vi "Retrieve All Paragraphs.vi"(8 "error in (no error)":errorcluster, 11 "xwpfReader in":refnum<class "xwpfReader.lvclass">) -> (0 "error out":errorcluster, 1 "Paragraph Styles":refnum<class "Style.lvclass">[](array[class]), 2 "Paragraphs":string[](array[string]), 3 "xwpfReader out":refnum<class "xwpfReader.lvclass">)   [LabVIEW 2017, in "LabVIEW NPOI.lvlib" / "xwpfReader.lvclass"]
doc: "Retrieves all the Paragraph content from the document. \n\nThis VI iterates through each paragraph to get their contents."
uses:
  xwpfReader.lvclass
  Styles/Style/Style.lvclass
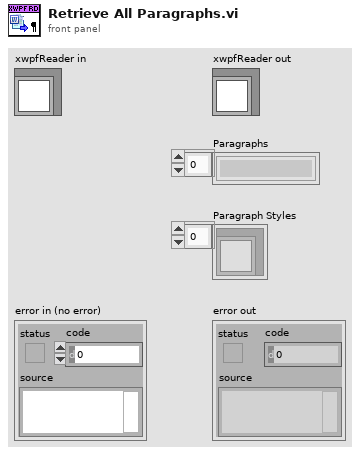
[diagram p1: front panel]
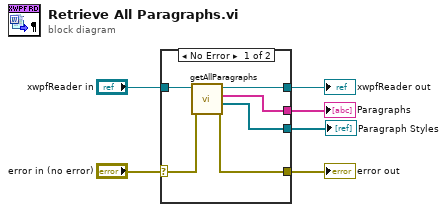
[diagram p0: block diagram]
diagram:
  n1 = case shown="No Error" "error in (no error)" {
    selector: "error in (no error)" -> [w10 w14]
    tunnel: [w9 w14] -> w5
    tunnel: [w11 w13] -> w3
    tunnel: "xwpfReader in" -> [w12 w13]
    tunnel: [w8 _] -> w2
    tunnel: [w7 _] -> w1
    frame No Error {
      n2 = call "getAllParagraphs.vi"("error in (no error)"=w10, "xwpfReader in"=w12) -> ("error out"=w9:errorcluster, "Paragraph Styles"=w7:refnum<class "Style.lvclass">[], "Paragraphs"=w8:string[], "xwpfReader out"=w11:refnum<class "xwpfReader.lvclass">)  [unwired: 6 in]
    }
    frame Error {
    }
  }
  "error out" <- w5
  "xwpfReader out" <- w3
  "Paragraphs" <- w2
  "Paragraph Styles" <- w1
